vi "Binary Stream Reader.vi"(8 "error in (no error)":errorcluster, 9 ".NET AdsBinaryReader refnum":refnum<k24>, 10 "Type":variant, 11 "TwinCAT ADS in":refnum<class "TwinCAT ADS.lvclass">) -> (0 "error out":errorcluster, 1 ".NET AdsBinaryReader refnum":refnum<k24>, 2 "Value":variant, 3 "TwinCAT ADS out":refnum<class "TwinCAT ADS.lvclass">)   [LabVIEW 2018, in "TwinCAT ADS.lvclass"]
uses:
  TwinCAT ADS.lvclass
  TwinCAT.Ads
  <vilib>/Utility/Data Type/NI_Data Type.lvlib
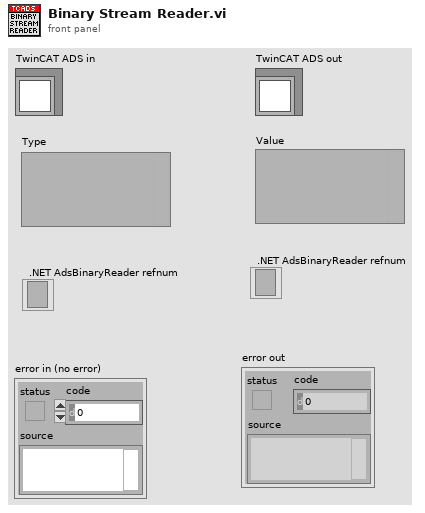
[diagram p1: front panel]
types:
  T1 = typedef "NI_Data Type.lvlib/Data Type.ctl" = enum8{"Invalid Type", "Void", "I8", "I16", "I32", "I64", "U8", "U16", "U32", "U64", "Single Float", "Double Float", "Extended Float", "Single Complex", "Double Complex", "Extended Complex", "Enum U8", "Enum U16", "Enum U32", "Enum U64", "Single Float With Unit", "Double Float With Unit", "Extended Float With Unit", "Single Complex with Unit", "Double Complex with Unit", "Extended Complex with Unit", "Boolean", "String", "Path", "Picture", "Tag", "Array", "Cluster", "Variant", "LV Variant", "Waveform", "Timestamp", "Digital Waveform", "Digital Data", "ExpressData", "Refnum", "External Data", "VI", "Poly VI", "LabVIEW Class Instance", "Fixed Point"}
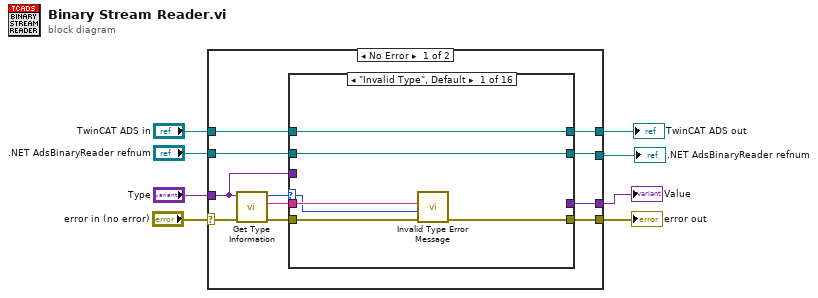
[diagram p0: block diagram]
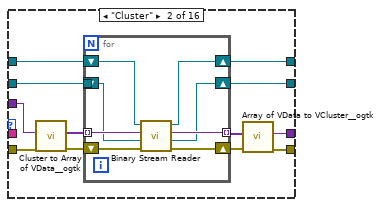
[diagram p2: hidden frame]
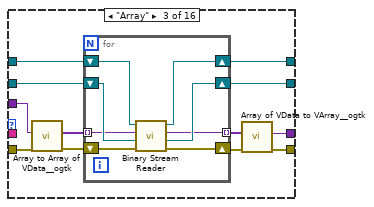
[diagram p3: hidden frame]
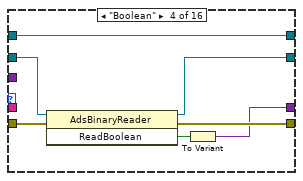
[diagram p4: hidden frame]
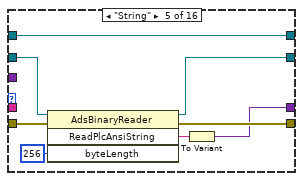
[diagram p5: hidden frame]
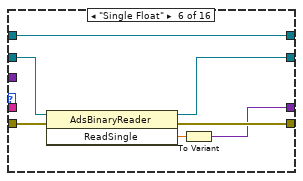
[diagram p6: hidden frame]
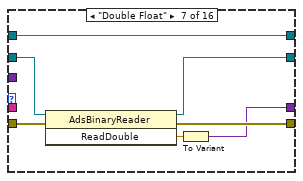
[diagram p7: hidden frame]
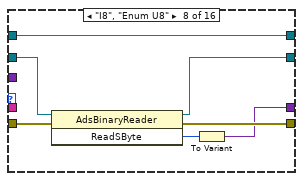
[diagram p8: hidden frame]
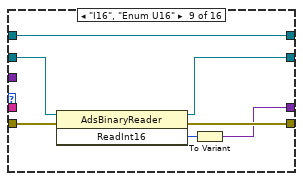
[diagram p9: hidden frame]
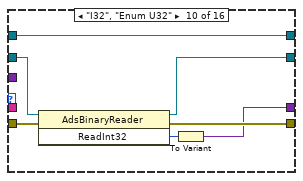
[diagram p10: hidden frame]
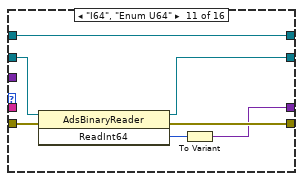
[diagram p11: hidden frame]
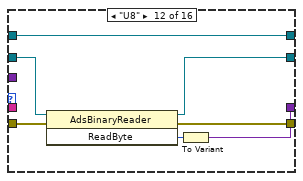
[diagram p12: hidden frame]
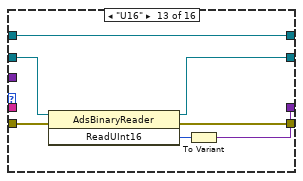
[diagram p13: hidden frame]
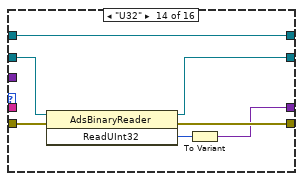
[diagram p14: hidden frame]
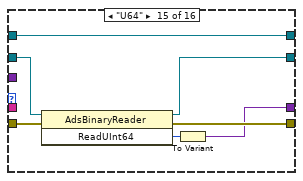
[diagram p15: hidden frame]
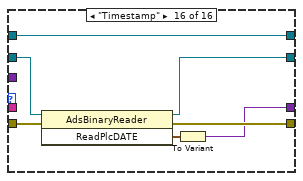
[diagram p16: hidden frame]
diagram:
  n1 = case shown="No Error" "error in (no error)" {
    selector: "error in (no error)" -> [w14 w160]
    tunnel: [w11 w160] -> w7
    tunnel: [w13 w159] -> w5
    tunnel: "TwinCAT ADS in" -> [w16 w159]
    tunnel: "Type" -> [w10 _]
    tunnel: ".NET AdsBinaryReader refnum" -> [w17 w158]
    tunnel: [w15 w158] -> w2
    tunnel: [w12 _] -> w1
    frame No Error {
      n2 = call <vilib>:"Get Type Information.vi"("error in (no error)"=w14, "Variant"=w10) -> ("error out"=w19:errorcluster, "Name"=w9:string, "Type"=w18:T1)  [unwired: 5 in, 2 out]
      n3 = case shown="\"Invalid Type\", Default" w18 {
        selector: w18 -> [w20 _ _ _ _ _ _ _ _ _ _ _ _ _ _ _]
        tunnel: w17 -> [w24 w34 w57 w72 w80 w87 w94 w101 w108 w115 w122 w129 w136 w143 w150 w157]
        tunnel: [w21 w27 w46 w71 w79 w86 w93 w100 w107 w114 w121 w128 w135 w142 w149 w156] -> w11
        tunnel: w19 -> [w23 w37 w54 w69 w77 w83 w91 w98 w105 w112 w119 w126 w133 w140 w147 w154]
        tunnel: w16 -> [w25 w33 w56 w70 w78 w85 w92 w99 w106 w113 w120 w127 w134 w141 w148 w155]
        tunnel: [w25 w32 w55 w70 w78 w85 w92 w99 w106 w113 w120 w127 w134 w141 w148 w155] -> w13
        tunnel: [_ w28 w49 w67 w76 w81 w89 w96 w102 w109 w117 w124 w130 w137 w144 w151] -> w12
        tunnel: [w24 w31 w50 w66 w74 w84 w88 w95 w104 w111 w116 w123 w132 w139 w146 w153] -> w15
        tunnel: w10 -> [_ w26 w51 _ _ _ _ _ _ _ _ _ _ _ _ _]
        tunnel: w9 -> [w22 _ _ _ _ _ _ _ _ _ _ _ _ _ _ _]
        frame "Invalid Type", Default {
          n4 = call "Invalid Type Error Message.vi"("error in (no error)"=w23, "Type"=w20, "Name"=w22) -> ("error out"=w21:errorcluster)  [unwired: 7 in, 1 out]
        }
        frame "Cluster" {
          n5 = call <userlib>:"Cluster to Array of VData__ogtk.vi"("error in (no error)"=w37, "Cluster"=w26) -> ("error out"=w36:errorcluster, "Array of VData"=w35:variant[])  [unwired: 8 in]
          n6 = for {
            shift-right: [w44] -> w30
            shift-left: w36 -> [w45]
            tunnel: w35 -> [w43] mode=indexing
            tunnel: w34 -> [w41]
            shift-right: [w39] -> w32
            shift-left: w33 -> [w42]
            tunnel: [w40] -> w29 mode=indexing
            shift-right: [w38] -> w31
            shift-left: _ -> [_]
            n7 = call "Binary Stream Reader.vi"("error in (no error)"=w45, ".NET AdsBinaryReader refnum"=w41, "Type"=w43, "TwinCAT ADS in"=w42) -> ("error out"=w44:errorcluster, ".NET AdsBinaryReader refnum"=w38:refnum<k24>, "Value"=w40:variant, "TwinCAT ADS out"=w39:refnum<class "TwinCAT ADS.lvclass">)  [unwired: 4 in]
          }
          n8 = call <userlib>:"Array of VData to VCluster__ogtk.vi"("error in (no error)"=w30, "Array"=w29) -> ("error out"=w27:errorcluster, "VCluster"=w28:variant)  [unwired: 8 in]
        }
        frame "Array" {
          n9 = call <userlib>:"Array to Array of VData__ogtk.vi"("error in (no error)"=w54, "MultiD Array"=w51) -> ("error out"=w53:errorcluster, "1D Array of Variants"=w52:variant[])  [unwired: 8 in]
          n10 = for {
            shift-right: [w64] -> w47
            shift-left: w53 -> [w65]
            tunnel: w52 -> [w59] mode=indexing
            shift-right: [w61] -> w55
            shift-left: w56 -> [w62]
            shift-right: [w60] -> w50
            shift-left: w57 -> [w63]
            tunnel: [w58] -> w48 mode=indexing
            n11 = call "Binary Stream Reader.vi"("error in (no error)"=w65, ".NET AdsBinaryReader refnum"=w63, "Type"=w59, "TwinCAT ADS in"=w62) -> ("error out"=w64:errorcluster, ".NET AdsBinaryReader refnum"=w60:refnum<k24>, "Value"=w58:variant, "TwinCAT ADS out"=w61:refnum<class "TwinCAT ADS.lvclass">)  [unwired: 4 in]
          }
          n12 = call <userlib>:"Array of VData to VArray__ogtk.vi"("error in (no error)"=w47, "1D Array of VData"=w48) -> ("error out"=w46:errorcluster, "VArray"=w49:variant)  [unwired: 8 in]
        }
        frame "Boolean" {
          n13 = invoke class="AdsBinaryReader" method="ReadBoolean"(reference=w72, error in=w69) -> (reference out=w66:refnum<k24>, error out=w71:errorcluster, "ReadBoolean"=w68:bool)  [unwired: 1 in]
          n14 = To Variant(anything=w68) -> (Variant=w67:variant)
        }
        frame "String" {
          n15 = invoke class="AdsBinaryReader" method="ReadPlcAnsiString"(reference=w80, error in=w77, "byteLength"=256) -> (reference out=w74:refnum<k24>, error out=w79:errorcluster, "ReadPlcAnsiString"=w75:string)  [unwired: 1 in, 1 out]
          n16 = To Variant(anything=w75) -> (Variant=w76:variant)
        }
        frame "Single Float" {
          n17 = invoke class="AdsBinaryReader" method="ReadSingle"(reference=w87, error in=w83) -> (reference out=w84:refnum<k24>, error out=w86:errorcluster, "ReadSingle"=w82:sgl)  [unwired: 1 in]
          n18 = To Variant(anything=w82) -> (Variant=w81:variant)
        }
        frame "Double Float" {
          n19 = invoke class="AdsBinaryReader" method="ReadDouble"(reference=w94, error in=w91) -> (reference out=w88:refnum<k24>, error out=w93:errorcluster, "ReadDouble"=w90:dbl)  [unwired: 1 in]
          n20 = To Variant(anything=w90) -> (Variant=w89:variant)
        }
        frame "I8", "Enum U8" {
          n21 = invoke class="AdsBinaryReader" method="ReadSByte"(reference=w101, error in=w98) -> (reference out=w95:refnum<k24>, error out=w100:errorcluster, "ReadSByte"=w97:i8)  [unwired: 1 in]
          n22 = To Variant(anything=w97) -> (Variant=w96:variant)
        }
        frame "I16", "Enum U16" {
          n23 = invoke class="AdsBinaryReader" method="ReadInt16"(reference=w108, error in=w105) -> (reference out=w104:refnum<k24>, error out=w107:errorcluster, "ReadInt16"=w103:i16)  [unwired: 1 in]
          n24 = To Variant(anything=w103) -> (Variant=w102:variant)
        }
        frame "I32", "Enum U32" {
          n25 = invoke class="AdsBinaryReader" method="ReadInt32"(reference=w115, error in=w112) -> (reference out=w111:refnum<k24>, error out=w114:errorcluster, "ReadInt32"=w110:i32)  [unwired: 1 in]
          n26 = To Variant(anything=w110) -> (Variant=w109:variant)
        }
        frame "I64", "Enum U64" {
          n27 = invoke class="AdsBinaryReader" method="ReadInt64"(reference=w122, error in=w119) -> (reference out=w116:refnum<k24>, error out=w121:errorcluster, "ReadInt64"=w118:i64)  [unwired: 1 in]
          n28 = To Variant(anything=w118) -> (Variant=w117:variant)
        }
        frame "U8" {
          n29 = invoke class="AdsBinaryReader" method="ReadByte"(reference=w129, error in=w126) -> (reference out=w123:refnum<k24>, error out=w128:errorcluster, "ReadByte"=w125:u8)  [unwired: 1 in]
          n30 = To Variant(anything=w125) -> (Variant=w124:variant)
        }
        frame "U16" {
          n31 = invoke class="AdsBinaryReader" method="ReadUInt16"(reference=w136, error in=w133) -> (reference out=w132:refnum<k24>, error out=w135:errorcluster, "ReadUInt16"=w131:u16)  [unwired: 1 in]
          n32 = To Variant(anything=w131) -> (Variant=w130:variant)
        }
        frame "U32" {
          n33 = invoke class="AdsBinaryReader" method="ReadUInt32"(reference=w143, error in=w140) -> (reference out=w139:refnum<k24>, error out=w142:errorcluster, "ReadUInt32"=w138:u32)  [unwired: 1 in]
          n34 = To Variant(anything=w138) -> (Variant=w137:variant)
        }
        frame "U64" {
          n35 = invoke class="AdsBinaryReader" method="ReadUInt64"(reference=w150, error in=w147) -> (reference out=w146:refnum<k24>, error out=w149:errorcluster, "ReadUInt64"=w145:u64)  [unwired: 1 in]
          n36 = To Variant(anything=w145) -> (Variant=w144:variant)
        }
        frame "Timestamp" {
          n37 = invoke class="AdsBinaryReader" method="ReadPlcDATE"(reference=w157, error in=w154) -> (reference out=w153:refnum<k24>, error out=w156:errorcluster, "ReadPlcDATE"=w152:timestamp)  [unwired: 1 in]
          n38 = To Variant(anything=w152) -> (Variant=w151:variant)
        }
      }
    }
    frame Error {
    }
  }
  "error out" <- w7
  "TwinCAT ADS out" <- w5
  ".NET AdsBinaryReader refnum" <- w2
  "Value" <- w1
